vi "Funkcja korelacji dla zakresu m.vi"(10 "Wyjscie 2":dbl[](array[numeric]), 11 "Wyjscie":dbl[](array[numeric])) -> (1 "Rxy":dbl[](array[numeric]), 2 "Wykres":cluster{i32[], dbl[]}, 3 "m":dbl[](array[numeric]))   [LabVIEW 2019]
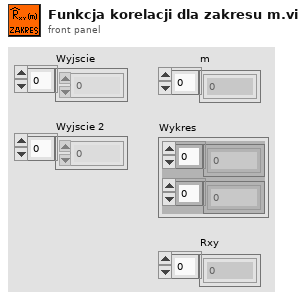
[diagram p1: front panel]
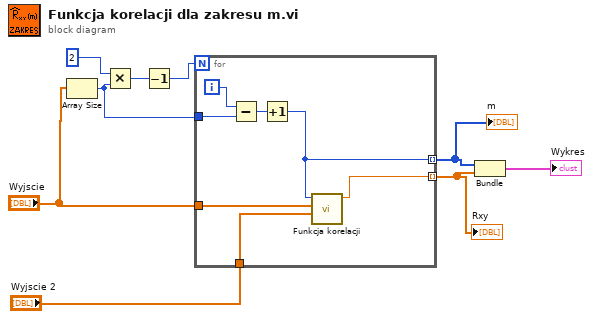
[diagram p0: block diagram]
diagram:
  n1 = Array Size(array="Wyjscie") -> (size(s)=w4:i32)
  n2 = Multiply(x=2, y=w4) -> (x*y=w2:i32)
  n3 = Decrement(x=w2) -> (x-1=w3:i32)
  n4 = for {
    N: w3 -> [_]
    tunnel: w4 -> [w15]
    tunnel: "Wyjscie" -> [w13]
    tunnel: "Wyjscie 2" -> [w12]
    tunnel: [w11] -> w9 mode=indexing
    tunnel: [w10] -> w8 mode=indexing
    i -> [w16]
    n5 = Subtract(x=w16, y=w15) -> (x-y=w14:i32)
    n6 = Increment(x=w14) -> (x+1=w10:i32)
    n7 = call "Funkcja korelacji.vi"("Sygnal 2"=w12, "Sygnal 1"=w13, "m"=w10) -> ("Funkcja korelacji"=w11:dbl)  [unwired: 8 in]
  }
  "m" <- w8
  "Rxy" <- w9
  n8 = Bundle(w8, w9) -> (→"Wykres":cluster{i32[], dbl[]})  [unwired: 1 in]
